vi "UseUSBAddress.vi"() -> ()   [LabVIEW 2009]
uses:
  C:/Samples/LabVIEW/UseUSBAddress/LabVIEW 2009/UsbDllWrap.dll
panel:
  out "Output:":string
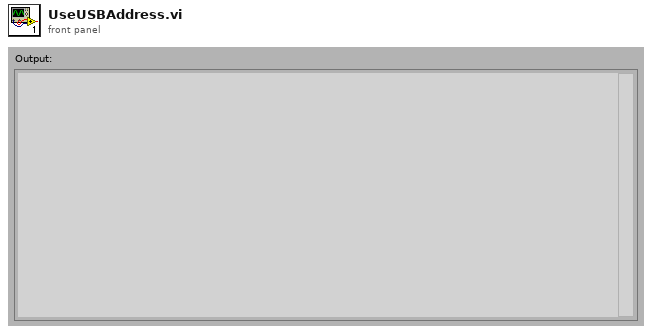
[diagram p1: front panel]
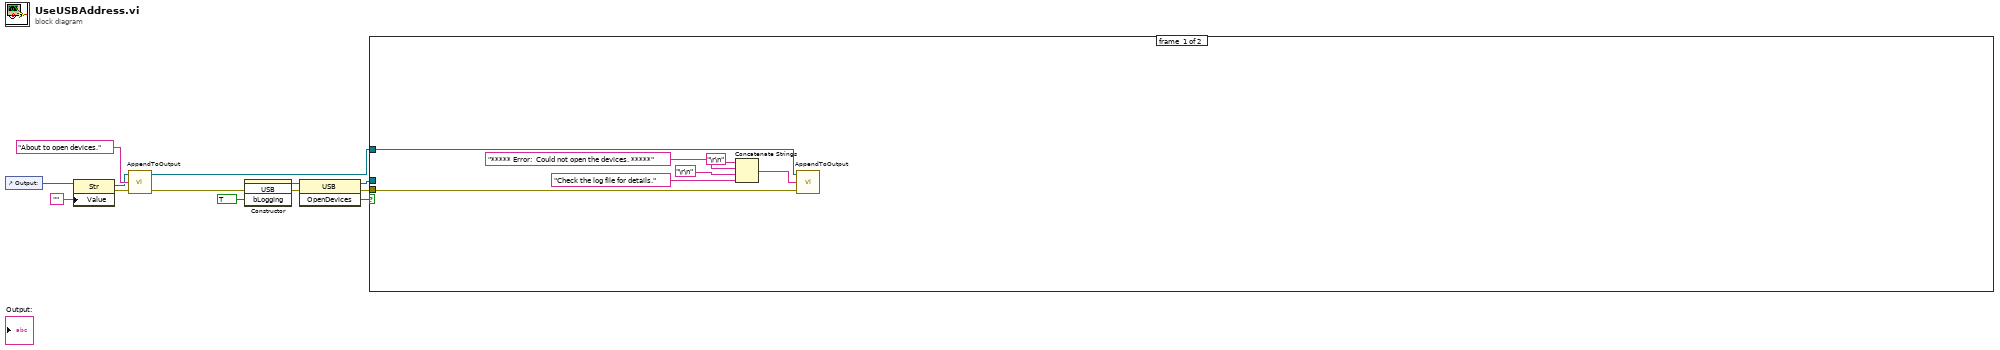
[diagram p0: block diagram]
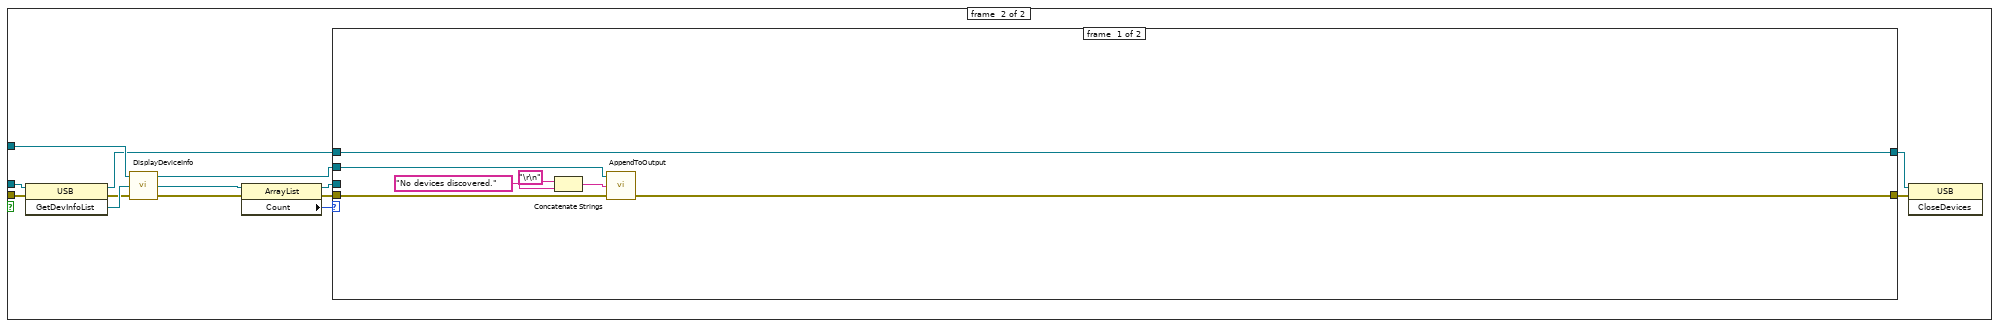
[diagram p2: hidden frame]
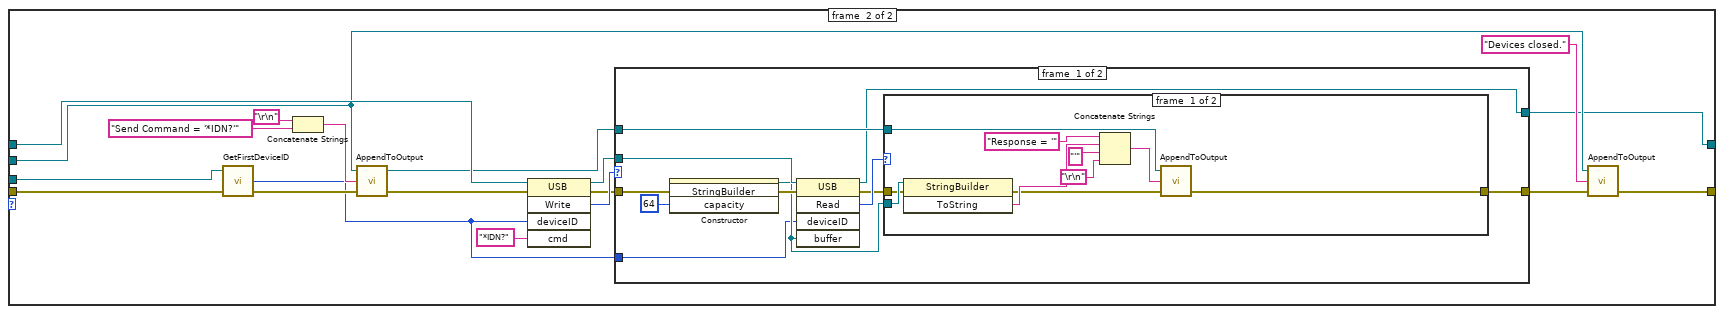
[diagram p3: hidden frame]
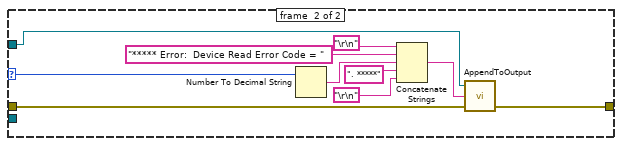
[diagram p4: hidden frame]
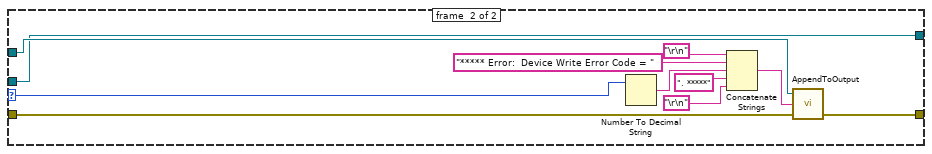
[diagram p5: hidden frame]
diagram:
  n1 = control-ref of="Output:"() -> (w4:refnum<vi>)
  n2 = property class="Str"(reference=w4, "Value"="") -> (reference out=w1:refnum<vi>, error out=w2:errorcluster)  [unwired: 1 in]
  n3 = call "AppendToOutput.vi"("error in"=w2, "Input String"="About to open devices.", "Output Refnum In"=w1) -> ("error out"=w11:errorcluster, "Output Refnum Out"=w8:refnum<vi>)  [unwired: 1 in]
  n4 = constructor class="USB"(error in=w11, "bLogging"=TRUE) -> (reference out=w10:refnum<k24>, error out=w7:errorcluster)  [unwired: 2 in, 2 out]
  n5 = invoke class="USB" method="OpenDevices"(reference=w10, error in=w7) -> (reference out=w5:refnum<k24>, error out=w6:errorcluster, "OpenDevices"=w9:bool)  [unwired: 1 in]
  n6 = case shown="True" w9 {
    tunnel: w8 -> [w20 w32]
    tunnel: w6 -> [w19 w33]
    tunnel: w5 -> [_ w34]
    frame #0 {
      n7 = Concatenate Strings("\r\n", "***** Error:  Could not open the devices. *****", "\r\n", "Check the log file for details.") -> (w15:string)
      n8 = call "AppendToOutput.vi"("error in"=w19, "Input String"=w15, "Output Refnum In"=w20) -> ()  [unwired: 1 in, 2 out]
    }
    frame #1 {
      n9 = invoke class="USB" method="GetDevInfoList"(reference=w34, error in=w33) -> (reference out=w29:refnum<k24>, error out=w30:errorcluster, "GetDevInfoList"=w31:refnum<k24>)  [unwired: 1 in]
      n10 = call "DisplayDeviceInfo.vi"("error in"=w30, "DevInfoList In"=w31, "Output Refnum In"=w32) -> ("error out"=w23:errorcluster, "DevInfoList Out"=w25:refnum<k24>, "Output Refnum Out"=w28:refnum<vi>)
      n11 = property class="ArrayList"(reference=w25, error in=w23) -> (reference out=w24:refnum<k24>, error out=w22:errorcluster, "Count"=w21:i32)
      n12 = case shown="0" w21 {
        tunnel: w29 -> [w39 w56]
        tunnel: w22 -> [w41 w54]
        tunnel: w24 -> [_ w53]
        tunnel: w28 -> [w38 w46]
        tunnel: [w40 w43] -> w27
        tunnel: [w39 w42] -> w26
        frame #0 {
          n13 = Concatenate Strings("\r\n", "No devices discovered." ("string")) -> (w35:string)
          n14 = call "AppendToOutput.vi"("error in"=w41, "Input String"=w35, "Output Refnum In"=w38) -> ("error out"=w40:errorcluster)  [unwired: 1 in, 1 out]
        }
        frame #1 {
          n15 = call "GetFirstDeviceID.vi"("error in"=w54, "DevInfoList In"=w53) -> ("error out"=w52:errorcluster, "Device ID"=w44:i32)  [unwired: 1 in, 1 out]
          n16 = Concatenate Strings("\r\n", "Send Command = '*IDN?'") -> (w58:string)
          n17 = call "AppendToOutput.vi"("error in"=w52, "Input String"=w58, "Output Refnum In"=w46) -> ("error out"=w55:errorcluster, "Output Refnum Out"=w48:refnum<vi>)  [unwired: 1 in]
          n18 = invoke class="USB" method="Write"(reference=w56, error in=w55, "deviceID"=w44, "cmd"="*IDN?") -> (reference out=w50:refnum<k24>, error out=w49:errorcluster, "Write"=w51:i32)  [unwired: 1 in, 2 out]
          n19 = case shown="0" w51 {
            selector: w51 -> [_ w97]
            tunnel: w50 -> [w71 w92]
            tunnel: w49 -> [w68 w95]
            tunnel: [w64 w94] -> w45
            tunnel: w48 -> [w63 w93]
            tunnel: w44 -> [w62 _]
            tunnel: [w61 w92] -> w42
            frame #0 {
              n20 = constructor class="StringBuilder"(error in=w68, "capacity"=64) -> (reference out=w66:refnum<k24>, error out=w69:errorcluster)  [unwired: 2 in, 2 out]
              n21 = invoke class="USB" method="Read"(reference=w71, error in=w69, "deviceID"=w62, "buffer"=w66) -> (reference out=w61:refnum<k24>, error out=w65:errorcluster, "Read"=w67:i32)  [unwired: 1 in, 2 out]
              n22 = case shown="0" w67 {
                selector: w67 -> [_ w86]
                tunnel: w66 -> [w81 _]
                tunnel: w65 -> [w80 w83]
                tunnel: [w73 w82] -> w64
                tunnel: w63 -> [w72 w84]
                frame #0 {
                  n23 = invoke class="StringBuilder" method="ToString"(reference=w81, error in=w80) -> (error out=w74:errorcluster, "ToString"=w77:string)  [unwired: 1 in, 1 out]
                  n24 = Concatenate Strings("Response = '", w77, "'", "\r\n") -> (w75:string)
                  n25 = call "AppendToOutput.vi"("error in"=w74, "Input String"=w75, "Output Refnum In"=w72) -> ("error out"=w73:errorcluster)  [unwired: 1 in, 1 out]
                }
                frame #1 {
                  n26 = Number To Decimal String(number=w86) -> (decimal integer string=w91:string)  [unwired: 1 in]
                  n27 = Concatenate Strings("\r\n", "***** Error:  Device Read Error Code = ", w91, ". *****", "\r\n") -> (w85:string)
                  n28 = call "AppendToOutput.vi"("error in"=w83, "Input String"=w85, "Output Refnum In"=w84) -> ("error out"=w82:errorcluster)  [unwired: 1 in, 1 out]
                }
              }
            }
            frame #1 {
              n29 = Number To Decimal String(number=w97) -> (decimal integer string=w98:string)  [unwired: 1 in]
              n30 = Concatenate Strings("\r\n", "***** Error:  Device Write Error Code = ", w98, ". *****", "\r\n") -> (w96:string)
              n31 = call "AppendToOutput.vi"("error in"=w95, "Input String"=w96, "Output Refnum In"=w93) -> ("error out"=w94:errorcluster)  [unwired: 1 in, 1 out]
            }
          }
          n32 = call "AppendToOutput.vi"("error in"=w45, "Input String"="Devices closed." ("string"), "Output Refnum In"=w46) -> ("error out"=w43:errorcluster)  [unwired: 1 in, 1 out]
        }
      }
      n33 = invoke class="USB" method="CloseDevices"(reference=w26, error in=w27) -> ()  [unwired: 1 in, 3 out]
    }
  }
